vi "RGB U32 Color Byte Location Test.vi"() -> ()   [LabVIEW 2018]
panel:
  out "LL":u8
  out "LH":u8
  out "HL":u8
  out "HH":u8
  in  "Color Box":u32(colorbox)
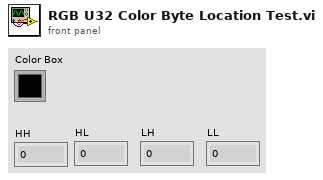
[diagram p1: front panel]
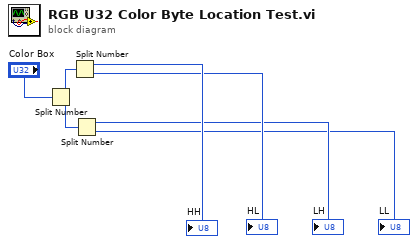
[diagram p0: block diagram]
diagram:
  n1 = Split Number(x="Color Box") -> (hi(x)=w5:u16, lo(x)=w6:u16)
  n2 = Split Number(x=w5) -> (hi(x)=→"HH":u8, lo(x)=→"HL":u8)
  n3 = Split Number(x=w6) -> (hi(x)=→"LH":u8, lo(x)=→"LL":u8)
